vi "move_picomotor.vi"(8 "error in":errorcluster, 9 "Destination (steps)":i16, 11 "Coarse Approach in":refnum<class "Coarse Approach.lvclass">) -> (0 "error out":errorcluster, 1 "Position (steps)":i32, 3 "Coarse Approach out":refnum<class "Coarse Approach.lvclass">)   [LabVIEW 2020, in "Coarse Approach.lvclass"]
uses:
  Coarse Approach.lvclass
  Coarse Approach.lvclass/Coarse Approach.ctl
  Picomotor/Picomotor.lvclass
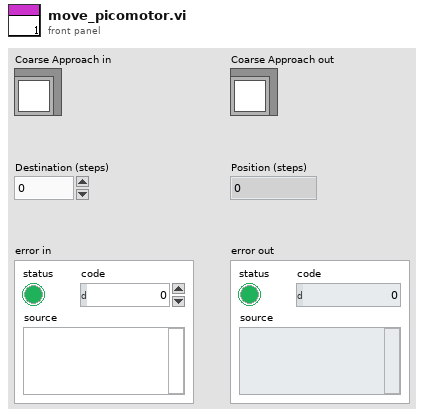
[diagram p1: front panel]
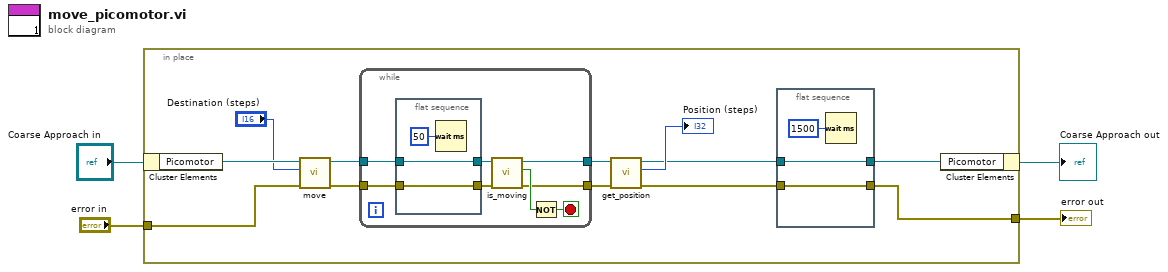
[diagram p0: block diagram]
diagram:
  n1 = in-place {
    in-place-border: "error in" -> [w12]
    in-place-border: [w5] -> w1
    n2 = in-place-cluster #1("Coarse Approach in") -> ("Picomotor"=w11:refnum<class "Picomotor.lvclass">)
    n3 = call-dynamic "move.vi"("error in"=w12, "Destination (steps)"="Destination (steps)", "Picomotor in"=w11) -> ("error out"=w15:errorcluster, "Picomotor out"=w16:refnum<class "Picomotor.lvclass">)  [unwired: 7 in]
    n4 = while {
      tunnel: w16 -> [w23]
      tunnel: w15 -> [w22]
      tunnel: [w25] -> w14
      tunnel: [w24] -> w13
      stop <- w26 stop-if-true
      n5 = flat-sequence {
        tunnel: w23 -> [w29]
        tunnel: w22 -> [w28]
        tunnel: [w29] -> w21
        tunnel: [w28] -> w20
        frame #0 {
          n6 = Wait (ms)(milliseconds to wait=u32 50) -> ()  [unwired: 1 out]
        }
      }
      n7 = call-dynamic "is_moving.vi"("error in (no error)"=w20, "Picomotor in"=w21) -> ("error out"=w24:errorcluster, "Is moving?"=w27:bool, "Picomotor out"=w25:refnum<class "Picomotor.lvclass">)  [unwired: 7 in]
      n8 = Not(x=w27) -> (.not. x?=w26:bool)
    }
    n9 = call-dynamic "get_position.vi"("error in"=w13, "Picomotor in"=w14) -> ("error out"=w7:errorcluster, "Position"=→"Position (steps)":i32, "Picomotor out"=w8:refnum<class "Picomotor.lvclass">)  [unwired: 7 in]
    n10 = flat-sequence {
      tunnel: w8 -> [w19]
      tunnel: w7 -> [w18]
      tunnel: [w19] -> w6
      tunnel: [w18] -> w5
      frame #0 {
        n11 = Wait (ms)(milliseconds to wait=u32 1500) -> ()  [unwired: 1 out]
      }
    }
    n12 = in-place-cluster #1("Picomotor"=w6) -> (→"Coarse Approach out":refnum<class "Coarse Approach.lvclass">)
  }
  "error out" <- w1
